vi "Packet_encode_TargetCornerArray.vi"(9 "TargetCornerArray":T1[](array[typedef]), 11 "RawData In":u8[](array[numeric])) -> (3 "RawData Out":u8[](array[numeric]))   [LabVIEW 2019, in "PhotonVisionLib.lvlib"]
doc: "Encode (or append) a Target Corner Array at the end of an array of bytes. No conversion is actually done, the memory is just copied to the end of the array.\n\nInputs\n - RawData In -- Array of bytes to be appended to..\n - Target Corner Array -- Array of Target Corner clusters to be encoded.\n\nOutputs\n - RawData Out -- Array of bytes containing the appended value."
uses:
  <vilib>/Rock Robotics/WPI/ThirdParty/JAS_Junk/TrajLib/VI/Transform3d_GetTranslation3d.vi
  <vilib>/Rock Robotics/WPI/ThirdParty/JAS_Junk/TrajLib/VI/Translation3d_GetXYZ.vi
  PhotonVisionLib.lvlib
  TypeDef/TargetCornerType.ctl
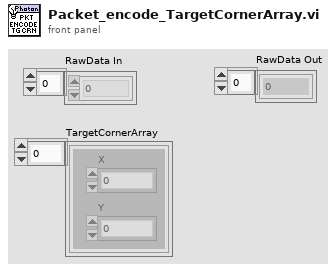
[diagram p1: front panel]
types:
  T1 = typedef "PhotonVisionLib.lvlib/TargetCornerType.ctl" = cluster{"X":dbl, "Y":dbl}
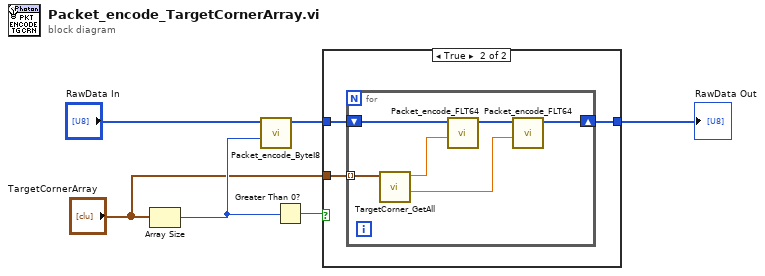
[diagram p0: block diagram]
diagram:
  n1 = Array Size(array="TargetCornerArray") -> (size(s)=w5:i32)
  n2 = call "Packet_encode_ByteI8.vi"("Int8_Value"=w5, "RawData In"="RawData In") -> ("RawData Out"=w2:u8[])  [unwired: 9 in]
  n3 = Greater Than 0?(x=w5) -> (x > 0?=w4:bool)
  n4 = case shown="True" w4 {
    tunnel: "TargetCornerArray" -> [_ w10]
    tunnel: w2 -> [w7 w9]
    tunnel: [w7 w8] -> w1
    frame False {
    }
    frame True {
      n5 = for {
        tunnel: w10 -> [w16] mode=indexing
        shift-right: [w13] -> w8
        shift-left: w9 -> [w14]
        n6 = call "TargetCorner_GetAll.vi"("TargetCorner"=w16) -> ("Y"=w11:dbl, "X"=w12:dbl)  [unwired: 9 in]
        n7 = call "Packet_encode_FLT64.vi"("FLT64_Value"=w12, "RawData In"=w14) -> ("RawData Out"=w15:u8[])  [unwired: 9 in]
        n8 = call "Packet_encode_FLT64.vi"("FLT64_Value"=w11, "RawData In"=w15) -> ("RawData Out"=w13:u8[])  [unwired: 9 in]
      }
    }
  }
  "RawData Out" <- w1
